vi "can decoder.vi"(10 "can cluster":T1 {"identifier" format="%03x"}, 11 "name":string="Prius") -> ()   [LabVIEW 2015]
uses:
  rio_Global.vi
panel:
  out "payload 2":u8[](array[numeric])
  out "payload":u8[](array[numeric])
  in  "sortbyID":bool
  in  "clear":bool
  out "can_log":u32[][](array[numeric]) format="%02x"
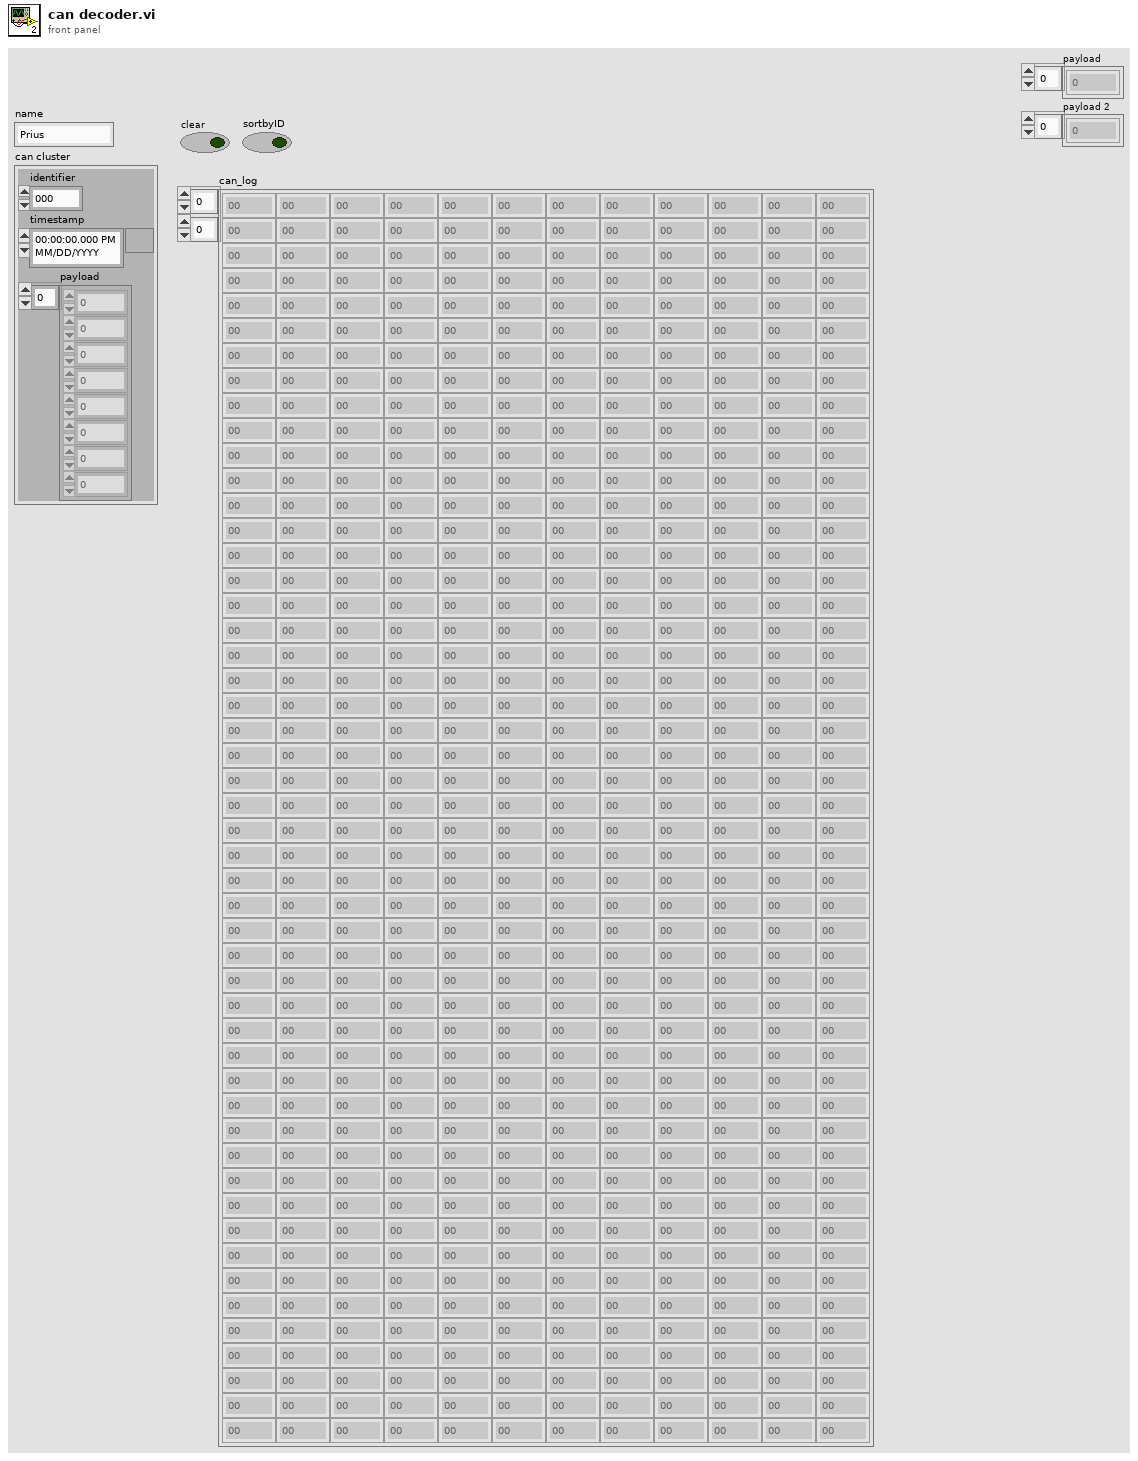
[diagram p1: front panel]
types:
  T1 = cluster{"identifier":u32, "timestamp":timestamp, "payload":u8[]}
  T2 = cluster{"identifier":u32, "identifier":u32, "identifier":u32, "identifier":u32, "identifier":u32, "identifier":u32, "identifier":u32, "identifier":u32, "identifier":u32, "identifier":u32, "identifier":u32}[]
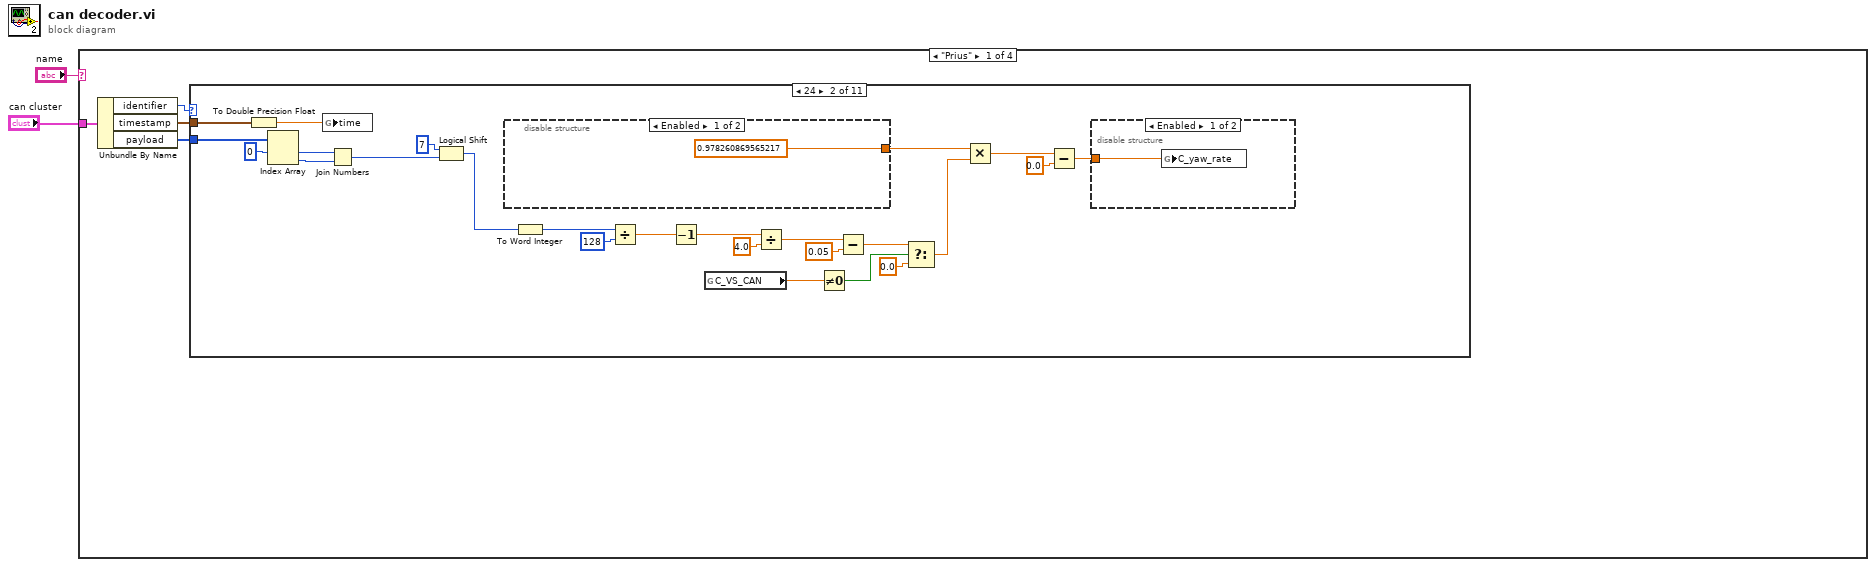
[diagram p0: block diagram]
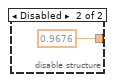
[diagram p3: hidden frame]
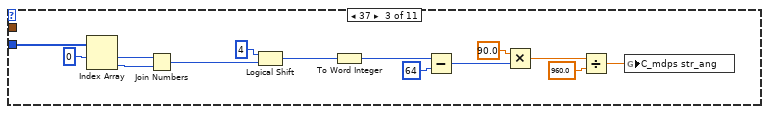
[diagram p5: hidden frame]
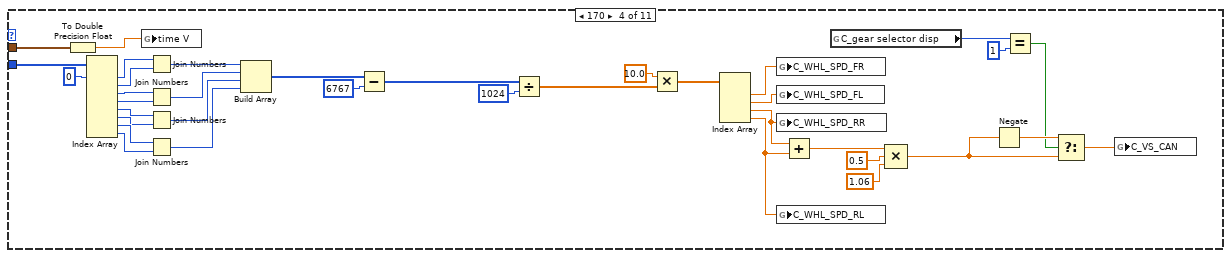
[diagram p6: hidden frame]
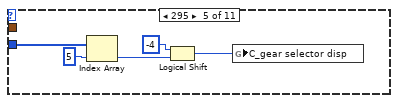
[diagram p7: hidden frame]
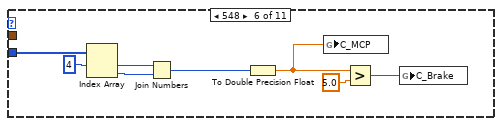
[diagram p8: hidden frame]
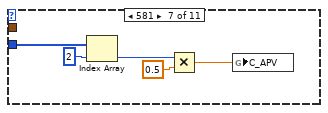
[diagram p9: hidden frame]
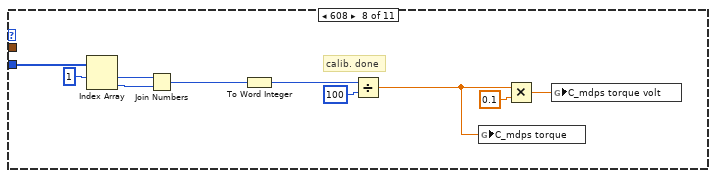
[diagram p10: hidden frame]
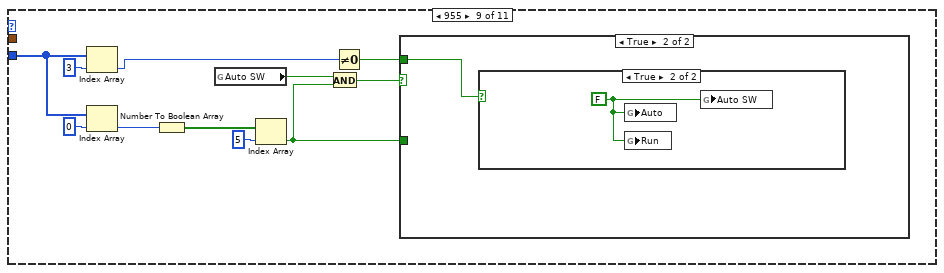
[diagram p11: hidden frame]
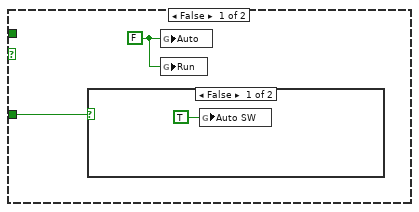
[diagram p12: hidden frame]
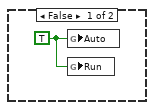
[diagram p14: hidden frame]
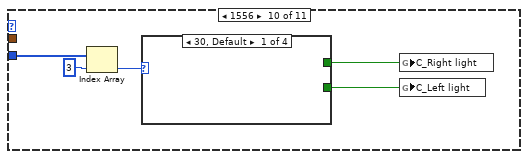
[diagram p15: hidden frame]
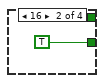
[diagram p16: hidden frame]
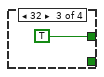
[diagram p17: hidden frame]
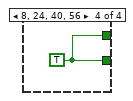
[diagram p18: hidden frame]
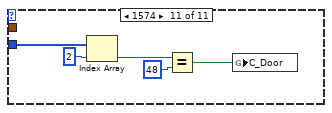
[diagram p19: hidden frame]
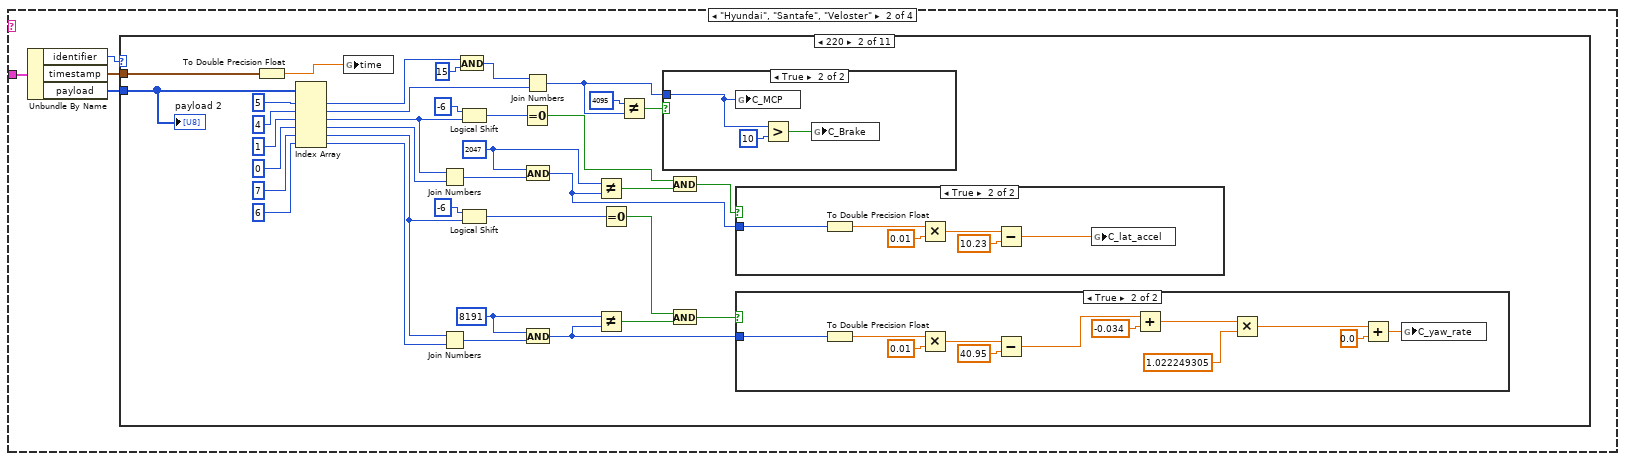
[diagram p20: hidden frame]
diagram:
  n1 = case shown="\"Prius\"" "name" {
    tunnel: "can cluster" -> [w6 w146 w412 w617]
    frame "Prius" {
      n2 = Unbundle By Name(w6) -> ("identifier"=w5:u32, "timestamp"=w4:timestamp, "payload"=w3:u8[])
      n3 = case shown="24" w5 {
        tunnel: w3 -> [_ w25 w41 w65 w89 w97 w102 w112 w115 w134 w142]
        tunnel: w4 -> [_ w22 _ w50 _ _ _ _ _ _ _]
        frame 0, Default {
        }
        frame 36 {
          n4 = To Double Precision Float(number=w22) -> (double precision float=w23:dbl)
          n5 = Index Array(array=w25, index #1=0 ("index")) -> (element #1=w27:u8, element #2=w19:u8)  [unwired: 1 in]
          n6 = global write "rio_Global.vi" "time"(w23) -> ()
          n7 = Join Numbers(hi=w27, lo=w19) -> ((hi.lo)=w18:u16)
          n8 = Logical Shift(y=i16 7, x=w18) -> (x << y=w31:u16)
          n9 = disable-structure shown="Enabled" {
            disable-tunnel: [0.978260869565217 ("x") 0.9676 ("x")] -> w8
            frame Enabled {
            }
            frame Disabled {
            }
          }
          n10 = To Word Integer(number=w31) -> (16bit integer=w30:i16)
          n11 = Divide(x=w30, y=i16 128) -> (x/y=w17:dbl)
          n12 = Decrement(x=w17) -> (x-1=w16:dbl)
          n13 = global read "rio_Global.vi" "C_VS_CAN"() -> (w13:dbl)
          n14 = Divide(x=w16, y=4.0) -> (x/y=w15:dbl)
          n15 = Not Equal To 0?(x=w13) -> (x != 0?=w12:bool)
          n16 = Subtract(x=w15, y=0.05) -> (x-y=w11:dbl)
          n17 = Select(t=w11, s=w12, f=0.0) -> (s? t:f=w9:dbl)
          n18 = Multiply(x=w8, y=w9) -> (x*y=w7:dbl)
          n19 = Subtract(x=w7, y=0.0) -> (x-y=w20:dbl)
          n20 = disable-structure shown="Enabled" {
            disable-tunnel: w20 -> [w34 _]
            frame Enabled {
              n21 = global write "rio_Global.vi" "C_yaw_rate"(w34) -> ()
            }
            frame Disabled {
            }
          }
        }
        frame 37 {
          n22 = Index Array(array=w41, index #1=0 ("index")) -> (element #1=w43:u8, element #2=w44:u8)  [unwired: 1 in]
          n23 = Join Numbers(hi=w43, lo=w44) -> ((hi.lo)=w45:u16)
          n24 = Logical Shift(y=i16 4, x=w45) -> (x << y=w47:u16)
          n25 = To Word Integer(number=w47) -> (16bit integer=w38:i16)
          n26 = Subtract(x=w38, y=i16 64) -> (x-y=w37:i16)
          n27 = Multiply(x=90.0, y=w37) -> (x*y=w39:dbl)
          n28 = Divide(x=w39, y=960.0) -> (x/y=w35:dbl)
          n29 = global write "rio_Global.vi" "C_mdps str_ang"(w35) -> ()
        }
        frame 170 {
          n30 = To Double Precision Float(number=w50) -> (double precision float=w49:dbl)
          n31 = Index Array(array=w65, index #1=0 ("index")) -> (element #1=w67:u8, element #2=w68:u8, element #3=w74:u8, element #4=w75:u8, element #5=w76:u8, element #6=w77:u8, element #7=w78:u8, element #8=w79:u8)  [unwired: 7 in]
          n32 = global write "rio_Global.vi" "time V"(w49) -> ()
          n33 = Join Numbers(hi=w67, lo=w68) -> ((hi.lo)=w80:u16)
          n34 = Join Numbers(hi=w74, lo=w75) -> ((hi.lo)=w81:u16)
          n35 = Join Numbers(hi=w76, lo=w77) -> ((hi.lo)=w82:u16)
          n36 = Join Numbers(hi=w78, lo=w79) -> ((hi.lo)=w83:u16)
          n37 = Build Array(w80, w81, w82, w83) -> (w84:u16[])
          n38 = Subtract(x=w84, y=u16 6767) -> (x-y=w70:u16[])
          n39 = Divide(x=w70, y=u16 1024) -> (x/y=w72:dbl[])
          n40 = Multiply(x=10.0, y=w72) -> (x*y=w64:dbl[])
          n41 = Index Array(array=w64) -> (element #1=w56:dbl, element #2=w57:dbl, element #3=w53:dbl, element #4=w52:dbl)  [unwired: 4 in]
          n42 = global write "rio_Global.vi" "C_WHL_SPD_FR"(w56) -> ()
          n43 = global write "rio_Global.vi" "C_WHL_SPD_FL"(w57) -> ()
          n44 = global write "rio_Global.vi" "C_WHL_SPD_RR"(w53) -> ()
          n45 = global write "rio_Global.vi" "C_WHL_SPD_RL"(w52) -> ()
          n46 = Add(x=w53, y=w52) -> (x+y=w63:dbl)
          n47 = global read "rio_Global.vi" "C_gear selector disp"() -> (w55:u8)
          n48 = Compound Arithmetic op=MULTIPLY(w63, 0.5 ("y"), 1.06 ("value")) -> (w58:dbl)
          n49 = Negate(x=w58) -> (-x=w61:dbl)
          n50 = Equal?(x=w55, y=u8 1) -> (x = y?=w60:bool)
          n51 = Select(t=w61, s=w60, f=w58) -> (s? t:f=w54:dbl)
          n52 = global write "rio_Global.vi" "C_VS_CAN"(w54) -> ()
        }
        frame 295 {
          n53 = Index Array(array=w89, index=5) -> (element=w86:u8)
          n54 = Logical Shift(y=i16 -4, x=w86) -> (x << y=w85:u8)
          n55 = global write "rio_Global.vi" "C_gear selector disp"(w85) -> ()
        }
        frame 548 {
          n56 = Index Array(array=w97, index #1=4 ("index")) -> (element #1=w95:u8, element #2=w94:u8)  [unwired: 1 in]
          n57 = Join Numbers(hi=w95, lo=w94) -> ((hi.lo)=w93:u16)
          n58 = To Double Precision Float(number=w93) -> (double precision float=w91:dbl)
          n59 = global write "rio_Global.vi" "C_MCP"(w91) -> ()
          n60 = Greater?(x=w91, y=5.0) -> (0:w90:bool)
          n61 = global write "rio_Global.vi" "C_Brake"(w90) -> ()
        }
        frame 581 {
          n62 = Index Array(array=w102, index=2) -> (element=w100:u8)
          n63 = Multiply(x=w100, y=0.5) -> (x*y=w98:dbl)
          n64 = global write "rio_Global.vi" "C_APV"(w98) -> ()
        }
        frame 608 {
          # "calib. done"
          n65 = Index Array(array=w112, index #1=1 ("index")) -> (element #1=w110:u8, element #2=w109:u8)  [unwired: 1 in]
          n66 = Join Numbers(hi=w110, lo=w109) -> ((hi.lo)=w108:u16)
          n67 = To Word Integer(number=w108) -> (16bit integer=w106:i16)
          n68 = Divide(x=w106, y=i16 100) -> (x/y=w104:dbl)
          n69 = global write "rio_Global.vi" "C_mdps torque"(w104) -> ()
          n70 = Multiply(x=w104, y=0.1) -> (x*y=w103:dbl)
          n71 = global write "rio_Global.vi" "C_mdps torque volt"(w103) -> ()
        }
        frame 955 {
          n72 = Index Array(array=w115, index=3) -> (element=w113:u8)
          n73 = Index Array(array=w115, index=0) -> (element=w122:u8)
          n74 = Number To Boolean Array(number=w122) -> (Boolean array=w121:bool[])
          n75 = global read "rio_Global.vi" "Auto SW"() -> (w119:bool)
          n76 = Index Array(array=w121, index=5) -> (element=w117:bool)
          n77 = And(x=w119, y=w117) -> (x .and. y?=w118:bool)
          n78 = Not Equal To 0?(x=w113) -> (x != 0?=w116:bool)
          n79 = case shown="True" w118 {
            tunnel: w116 -> [_ w127]
            tunnel: w117 -> [w125 _]
            frame False {
              w124 = FALSE ("Auto SW")
              n80 = case shown="False" w125 {
                frame False {
                  n81 = global write "rio_Global.vi" "Auto SW"(TRUE ("Auto SW")) -> ()
                }
                frame True {
                }
              }
              n82 = global write "rio_Global.vi" "Auto"(w124) -> ()
              n83 = global write "rio_Global.vi" "Run"(w124) -> ()
            }
            frame True {
              n84 = case shown="True" w127 {
                frame False {
                  w128 = TRUE ("Auto")
                  n85 = global write "rio_Global.vi" "Auto"(w128) -> ()
                  n86 = global write "rio_Global.vi" "Run"(w128) -> ()
                }
                frame True {
                  w129 = FALSE ("Auto SW")
                  n87 = global write "rio_Global.vi" "Auto"(w129) -> ()
                  n88 = global write "rio_Global.vi" "Run"(w129) -> ()
                  n89 = global write "rio_Global.vi" "Auto SW"(w129) -> ()
                }
              }
            }
          }
        }
        frame 1556 {
          n90 = Index Array(array=w134, index=3) -> (element=w132:u8)
          n91 = case shown="30, Default" w132 {
            tunnel: [_ TRUE _ w137] -> w131
            tunnel: [_ _ TRUE w137] -> w130
            frame 48, Default {
            }
            frame 16 {
            }
            frame 32 {
            }
            frame 8, 24, 40, 56 {
              w137 = TRUE
            }
          }
          n92 = global write "rio_Global.vi" "C_Right light"(w130) -> ()
          n93 = global write "rio_Global.vi" "C_Left light"(w131) -> ()
        }
        frame 1574 {
          n94 = Index Array(array=w142, index=2) -> (element=w140:u8)
          n95 = Equal?(x=w140, y=u8 48) -> (x = y?=w138:bool)
          n96 = global write "rio_Global.vi" "C_Door"(w138) -> ()
        }
      }
    }
    frame "Hyundai", "Santafe", "Veloster" {
      n97 = Unbundle By Name(w146) -> ("identifier"=w145:u32, "timestamp"=w144:timestamp, "payload"=w143:u8[])
      n98 = case shown="220" w145 {
        tunnel: w143 -> [_ w147 w205 w223 w244 w299 w303 w305 w314 w368 w392]
        tunnel: w144 -> [_ w182 _ _ _ _ _ _ w312 _ _]
        frame 0, Default {
        }
        frame 544 {
          w151 = u16 8191
          w158 = u16 2047
          n99 = To Double Precision Float(number=w182) -> (double precision float=w181:dbl)
          n100 = Index Array(array=w147, index #1=5 ("index"), index #2=4 ("index"), index #3=1 ("index"), index #4=0 ("index"), index #5=7 ("index"), index #6=6 ("index")) -> (element #1=w174:u8, element #2=w173:u8, element #3=w172:u8, element #4=w171:u8, element #5=w170:u8, element #6=w169:u8)
          n101 = global write "rio_Global.vi" "time"(w181) -> ()
          n102 = Join Numbers(hi=w172, lo=w171) -> ((hi.lo)=w159:u16)
          n103 = Join Numbers(hi=w170, lo=w169) -> ((hi.lo)=w150:u16)
          n104 = And(x=w174, y=u8 15) -> (x .and. y?=w167:u8)
          n105 = Logical Shift(y=i16 -6, x=w172) -> (x << y=w161:u8)
          n106 = Logical Shift(y=i16 -6, x=w170) -> (x << y=w154:u8)
          n107 = Equal To 0?(x=w161) -> (x = 0?=w162:bool)
          n108 = Join Numbers(hi=w167, lo=w173) -> ((hi.lo)=w164:u16)
          n109 = And(x=w158, y=w159) -> (x .and. y?=w157:u16)
          n110 = And(x=w151, y=w150) -> (x .and. y?=w149:u16)
          n111 = Not Equal?(x=w158, y=w157) -> (x != y?=w163:bool)
          n112 = Not Equal?(x=w151, y=w149) -> (x != y?=w152:bool)
          n113 = Equal To 0?(x=w154) -> (x = 0?=w153:bool)
          n114 = Not Equal?(x=u16 4095, y=w164) -> (x != y?=w165:bool)
          n115 = case shown="True" w165 {
            tunnel: w164 -> [_ w201]
            frame False {
            }
            frame True {
              n116 = global write "rio_Global.vi" "C_MCP"(w201) -> ()
              n117 = Greater?(x=w201, y=u16 10) -> (0:w203:bool)
              n118 = global write "rio_Global.vi" "C_Brake"(w203) -> ()
            }
          }
          n119 = And(x=w162, y=w163) -> (x .and. y?=w156:bool)
          n120 = And(x=w153, y=w152) -> (x .and. y?=w148:bool)
          n121 = case shown="True" w156 {
            tunnel: w157 -> [_ w200]
            frame False {
            }
            frame True {
              n122 = To Double Precision Float(number=w200) -> (double precision float=w199:dbl)
              n123 = Multiply(x=w199, y=0.01) -> (x*y=w197:dbl)
              n124 = Subtract(x=w197, y=10.23) -> (x-y=w195:dbl)
              n125 = global write "rio_Global.vi" "C_lat_accel"(w195) -> ()
            }
          }
          n126 = case shown="True" w148 {
            tunnel: w149 -> [_ w194]
            frame False {
            }
            frame True {
              n127 = To Double Precision Float(number=w194) -> (double precision float=w193:dbl)
              n128 = Multiply(x=w193, y=0.01) -> (x*y=w191:dbl)
              n129 = Subtract(x=w191, y=40.95) -> (x-y=w184:dbl)
              n130 = Add(x=w184, y=-0.034) -> (x+y=w183:dbl)
              n131 = Multiply(x=w183, y=1.022249305) -> (x*y=w187:dbl)
              n132 = Add(x=w187, y=0.0) -> (x+y=w186:dbl)
              n133 = global write "rio_Global.vi" "C_yaw_rate"(w186) -> ()
            }
          }
          "payload 2" <- w147
        }
        frame 608 {
          n134 = global read "rio_Global.vi" "Car_name"() -> (w204:string)
          n135 = Equal?(x=w204, y="Santafe") -> (x = y?=w206:bool)
          n136 = case shown="True" w206 {
            tunnel: w205 -> [_ w216]
            frame False {
            }
            frame True {
              n137 = Index Array(array=w216, index=3) -> (element=w214:u8)
              n138 = Number To Boolean Array(number=w214) -> (Boolean array=w213:bool[])
              n139 = global read "rio_Global.vi" "Auto SW"() -> (w210:bool)
              n140 = Index Array(array=w213, index #1=1 ("index")) -> (element #1=w208:bool, element #2=w211:bool)  [unwired: 1 in]
              n141 = And(x=w210, y=w208) -> (x .and. y?=w209:bool)
              n142 = case shown="False" w209 {
                tunnel: w211 -> [_ w220]
                tunnel: w208 -> [w218 _]
                frame False {
                  w217 = FALSE ("Auto SW")
                  n143 = case shown="False" w218 {
                    frame False {
                      n144 = global write "rio_Global.vi" "Auto SW"(TRUE ("Auto SW")) -> ()
                    }
                    frame True {
                    }
                  }
                  n145 = global write "rio_Global.vi" "Auto"(w217) -> ()
                  n146 = global write "rio_Global.vi" "Run"(w217) -> ()
                }
                frame True {
                  n147 = case shown="True" w220 {
                    frame False {
                      w221 = TRUE ("Auto")
                      n148 = global write "rio_Global.vi" "Auto"(w221) -> ()
                      n149 = global write "rio_Global.vi" "Run"(w221) -> ()
                    }
                    frame True {
                      w222 = FALSE ("Auto SW")
                      n150 = global write "rio_Global.vi" "Auto"(w222) -> ()
                      n151 = global write "rio_Global.vi" "Run"(w222) -> ()
                      n152 = global write "rio_Global.vi" "Auto SW"(w222) -> ()
                    }
                  }
                }
              }
            }
          }
        }
        frame 809 {
          n153 = Index Array(array=w223, index #1=5 ("index"), index #2=6 ("index")) -> (element #1=w226:u8, element #2=w229:u8)
          n154 = Not Equal?(x=w226, y=u8 255 ("x")) -> (x != y?=w230:bool)
          n155 = Not Equal?(x=w229, y=u8 255 ("x")) -> (x != y?=w231:bool)
          n156 = case shown="True" w230 {
            tunnel: w226 -> [_ w243]
            frame False {
            }
            frame True {
              n157 = Subtract(x=w243, y=u8 32) -> (x-y=w241:u8)
              n158 = To Double Precision Float(number=w241) -> (double precision float=w240:dbl)
              n159 = Multiply(x=w240, y=100.0) -> (x*y=w238:dbl)
              n160 = Divide(x=w238, y=213.0) -> (x/y=w236:dbl)
              n161 = global write "rio_Global.vi" "C_tps"(w236) -> ()
            }
          }
          n162 = case shown="True" w231 {
            tunnel: w229 -> [_ w235]
            frame False {
            }
            frame True {
              n163 = To Double Precision Float(number=w235) -> (double precision float=w234:dbl)
              n164 = Multiply(x=w234, y=0.3906) -> (x*y=w233:dbl)
              n165 = global write "rio_Global.vi" "C_APV"(w233) -> ()
            }
          }
        }
        frame 914 {
          n166 = Array Subset(array=w244, index=0, length=7) -> (w248:u8[])
          n167 = Index Array(array=w244, index #1=7 ("index"), index #2=2 ("index"), index #3=1 ("index"), index #4=4 ("index"), index #5=3 ("index")) -> (element #1=w245:u8, element #2=w256:u8, element #3=w255:u8, element #4=w252:u8, element #5=w251:u8)
          n168 = Add Array Elements(numeric array=w248) -> (sum=w246:u8)
          n169 = Equal?(x=w246, y=w245) -> (x = y?=w247:bool)
          n170 = case shown="True" w247 {
            tunnel: w256 -> [_ w270]
            tunnel: w255 -> [_ w269]
            tunnel: w252 -> [_ w266]
            tunnel: w251 -> [_ w265]
            frame False {
            }
            frame True {
              w261 = u16 4095 ("y")
              n171 = Join Numbers(hi=w270, lo=w269) -> ((hi.lo)=w262:u16)
              n172 = Join Numbers(hi=w266, lo=w265) -> ((hi.lo)=w267:u16)
              n173 = And(x=w261, y=w262) -> (x .and. y?=w260:u16)
              n174 = Not Equal?(x=w267, y=u16 32767 ("x")) -> (x != y?=w263:bool)
              n175 = Not Equal?(x=w261, y=w260) -> (x != y?=w264:bool)
              n176 = case shown="True" w264 {
                tunnel: w260 -> [_ w283]
                frame False {
                }
                frame True {
                  n177 = To Double Precision Float(number=w283) -> (double precision float=w282:dbl)
                  n178 = Subtract(x=w282, y=2048.0) -> (x-y=w281:dbl)
                  n179 = Multiply(x=w281, y=0.01) -> (x*y=w280:dbl)
                  n180 = global write "rio_Global.vi" "C_mdps torque"(w280) -> ()
                }
              }
              n181 = case shown="True" w263 {
                tunnel: w267 -> [_ w277]
                frame False {
                }
                frame True {
                  n182 = To Double Precision Float(number=w277) -> (double precision float=w274:dbl)
                  n183 = Subtract(x=w274, y=65536.0) -> (x-y=w275:dbl)
                  n184 = Greater?(x=w274, y=32767.0 ("x")) -> (0:w278:bool)
                  n185 = Select(t=w275, s=w278, f=w274) -> (s? t:f=w273:dbl)
                  n186 = Multiply(x=w273, y=0.1) -> (x*y=w271:dbl)
                  n187 = global write "rio_Global.vi" "C_mdps str_ang"(w271) -> ()
                }
              }
            }
          }
        }
        frame 688 {
          n188 = Index Array(array=w299, index #1=1 ("index"), index #2=0 ("index")) -> (element #1=w296:u8, element #2=w295:u8)
          n189 = Join Numbers(hi=w296, lo=w295) -> ((hi.lo)=w287:u16)
          n190 = To Long Integer(number=w287) -> (32bit integer=w286:i32)
          n191 = Greater?(x=w286, y=32767) -> (0:w293:bool)
          n192 = Subtract(x=w286, y=65535) -> (x-y=w291:i32)
          n193 = Select(t=w291, s=w293, f=w286) -> (s? t:f=w290:i32)
          n194 = Multiply(x=w290, y=0.1) -> (x*y=w288:dbl)
          n195 = disable-structure shown="Disabled" {
            disable-tunnel: w288 -> [w300 _]
            frame Disabled {
              n196 = global write "rio_Global.vi" "C_mdps str_ang"(w300) -> ()
            }
            frame Enabled {
            }
          }
        }
        frame 790 {
          n197 = Index Array(array=w303, index=6) -> (element=w301:u8)
          n198 = disable-structure shown="Disabled" {
            disable-tunnel: w301 -> [w304 _]
            frame Disabled {
              n199 = global write "rio_Global.vi" "C_VS_CAN"(w304) -> ()
            }
            frame Enabled {
            }
          }
        }
        frame 1087 {
          w308 = u8 15 ("y")
          n200 = Index Array(array=w305, index=1) -> (element=w307:u8)
          n201 = And(x=w307, y=w308) -> (x .and. y?=w309:u8)
          n202 = Not Equal?(x=w309, y=w308) -> (x != y?=w310:bool)
          n203 = case shown="True" w310 {
            tunnel: w309 -> [_ w311]
            frame False {
            }
            frame True {
              n204 = global write "rio_Global.vi" "C_gear selector disp"(w311) -> ()
            }
          }
        }
        frame 1200 {
          w318 = u16 16383 ("x")
          w331 = u16 16383 ("x")
          n205 = To Double Precision Float(number=w312) -> (double precision float=w313:dbl)
          n206 = Index Array(array=w314, index #1=1 ("index"), index #2=0 ("index"), index #3=3 ("index"), index #4=2 ("index"), index #5=5 ("index"), index #6=4 ("index"), index #7=7 ("index"), index #8=6 ("index")) -> (element #1=w323:u8, element #2=w322:u8, element #3=w321:u8, element #4=w320:u8, element #5=w341:u8, element #6=w340:u8, element #7=w336:u8, element #8=w335:u8)
          n207 = global write "rio_Global.vi" "time V"(w313) -> ()
          n208 = Join Numbers(hi=w323, lo=w322) -> ((hi.lo)=w319:u16)
          n209 = Join Numbers(hi=w321, lo=w320) -> ((hi.lo)=w317:u16)
          n210 = Join Numbers(hi=w341, lo=w340) -> ((hi.lo)=w339:u16)
          n211 = Join Numbers(hi=w336, lo=w335) -> ((hi.lo)=w332:u16)
          n212 = And(x=w319, y=w318) -> (x .and. y?=w316:u16)
          n213 = And(x=w318, y=w317) -> (x .and. y?=w315:u16)
          n214 = And(x=w339, y=w331) -> (x .and. y?=w330:u16)
          n215 = And(x=w331, y=w332) -> (x .and. y?=w329:u16)
          n216 = Not Equal?(x=w330, y=w331) -> (x != y?=w334:bool)
          n217 = Not Equal?(x=w331, y=w329) -> (x != y?=w333:bool)
          n218 = And(x=w334, y=w333) -> (x .and. y?=w328:bool)
          n219 = case shown="True" w328 {
            tunnel: w330 -> [_ w367]
            tunnel: w329 -> [_ w366]
            tunnel: w316 -> [_ w360]
            tunnel: w315 -> [_ w359]
            frame False {
            }
            frame True {
              w355 = 0.03125 ("y")
              w365 = 0.03125 ("y")
              n220 = To Double Precision Float(number=w360) -> (double precision float=w357:dbl)
              n221 = To Double Precision Float(number=w359) -> (double precision float=w354:dbl)
              n222 = To Double Precision Float(number=w367) -> (double precision float=w358:dbl)
              n223 = To Double Precision Float(number=w366) -> (double precision float=w351:dbl)
              n224 = Multiply(x=w357, y=w355) -> (x*y=w356:dbl)
              n225 = Multiply(x=w355, y=w354) -> (x*y=w353:dbl)
              n226 = Multiply(x=w358, y=w365) -> (x*y=w352:dbl)
              n227 = Multiply(x=w365, y=w351) -> (x*y=w350:dbl)
              n228 = global write "rio_Global.vi" "C_WHL_SPD_FL"(w356) -> ()
              n229 = global write "rio_Global.vi" "C_WHL_SPD_FR"(w353) -> ()
              n230 = global write "rio_Global.vi" "C_WHL_SPD_RL"(w352) -> ()
              n231 = global write "rio_Global.vi" "C_WHL_SPD_RR"(w350) -> ()
              n232 = Add(x=w352, y=w350) -> (x+y=w364:dbl)
              n233 = global read "rio_Global.vi" "C_gear selector disp"() -> (w347:u8)
              n234 = Multiply(x=w364, y=0.5) -> (x*y=w361:dbl)
              n235 = Multiply(x=w361, y=1.0) -> (x*y=w345:dbl)
              n236 = Negate(x=w345) -> (-x=w349:dbl)
              n237 = Equal?(x=w347, y=u8 7) -> (x = y?=w348:bool)
              n238 = Select(t=w349, s=w348, f=w345) -> (s? t:f=w344:dbl)
              n239 = global write "rio_Global.vi" "C_VS_CAN"(w344) -> ()
            }
          }
          "payload" <- w314
        }
        frame 1264 {
          n240 = disable-structure shown="Enabled" {
            disable-tunnel: w368 -> [w373 w377]
            frame Disabled {
              n241 = Index Array(array=w373, index=3) -> (element=w371:u8)
              n242 = case shown="8, 18, 28, 38" w371 {
                tunnel: [_ TRUE _ w376] -> w370
                tunnel: [_ _ TRUE w376] -> w369
                frame 48, Default {
                }
                frame 16 {
                }
                frame 32 {
                }
                frame 8, 24, 40, 56 {
                  w376 = TRUE
                }
              }
              n243 = global write "rio_Global.vi" "C_Right light"(w369) -> ()
              n244 = global write "rio_Global.vi" "C_Left light"(w370) -> ()
            }
            frame Enabled {
              n245 = Index Array(array=w377, index #1=7 ("index"), index #2=6 ("index"), index #3=5 ("index")) -> (element #1=w383:u8, element #2=w381:u8, element #3=w382:u8)
              n246 = Join Numbers(hi=w381, lo=w382) -> ((hi.lo)=w386:u16)
              n247 = Join Numbers(hi=u8 0, lo=w383) -> ((hi.lo)=w385:u16)
              n248 = Join Numbers(hi=w385, lo=w386) -> ((hi.lo)=w388:u32)
              n249 = Not Equal?(x=u32 16777215, y=w388) -> (x != y?=w389:bool)
              n250 = case shown="True" w389 {
                tunnel: w388 -> [_ w391]
                frame False {
                }
                frame True {
                  n251 = To Double Precision Float(number=w391) -> (double precision float=w390:dbl)
                  n252 = global write "rio_Global.vi" "C_odometer"(w390) -> ()
                }
              }
            }
          }
        }
        frame 1349 {
          n253 = disable-structure shown="Enabled" {
            disable-tunnel: w392 -> [w397 w398]
            frame Disabled {
              n254 = Index Array(array=w397, index=2) -> (element=w395:u8)
              n255 = Equal?(x=w395, y=u8 48) -> (x = y?=w393:bool)
              n256 = global write "rio_Global.vi" "C_Door"(w393) -> ()
            }
            frame Enabled {
              n257 = Index Array(array=w398, index=3) -> (element=w401:u8)
              n258 = Not Equal?(x=w401, y=u8 255 ("x")) -> (x != y?=w399:bool)
              n259 = case shown="True" w399 {
                tunnel: w401 -> [_ w408]
                frame False {
                }
                frame True {
                  n260 = To Double Precision Float(number=w408) -> (double precision float=w407:dbl)
                  n261 = Multiply(x=26.0, y=w407) -> (x*y=w405:dbl)
                  n262 = Divide(x=w405, y=256.0) -> (x/y=w403:dbl)
                  n263 = global write "rio_Global.vi" "C_battery voltage"(w403) -> ()
                }
              }
            }
          }
        }
      }
    }
    frame "Avante" {
      n264 = Unbundle By Name(w412) -> ("identifier"=w411:u32, "timestamp"=w410:timestamp, "payload"=w409:u8[])
      n265 = case shown="220" w411 {
        tunnel: w409 -> [_ w414 w477 w513 w514 w523 w577 w604]
        tunnel: w410 -> [_ w446 _ _ _ w521 _ _]
        frame 0, Default {
        }
        frame 544 {
          w417 = u16 8191
          w422 = u16 2047
          n266 = To Double Precision Float(number=w446) -> (double precision float=w445:dbl)
          n267 = Index Array(array=w414, index #1=4 ("index"), index #2=3 ("index"), index #3=1 ("index"), index #4=0 ("index"), index #5=6 ("index"), index #6=5 ("index")) -> (element #1=w438:u8, element #2=w437:u8, element #3=w436:u8, element #4=w435:u8, element #5=w434:u8, element #6=w433:u8)
          n268 = global write "rio_Global.vi" "time"(w445) -> ()
          n269 = Join Numbers(hi=w436, lo=w435) -> ((hi.lo)=w423:u16)
          n270 = Join Numbers(hi=w434, lo=w433) -> ((hi.lo)=w416:u16)
          n271 = And(x=w438, y=u8 15) -> (x .and. y?=w431:u8)
          n272 = Logical Shift(y=i16 -6, x=w436) -> (x << y=w425:u8)
          n273 = Logical Shift(y=i16 -6, x=w434) -> (x << y=w418:u8)
          n274 = Equal To 0?(x=w418) -> ()  [unwired: 1 out]
          n275 = Join Numbers(hi=w431, lo=w437) -> ((hi.lo)=w428:u16)
          n276 = Equal To 0?(x=w425) -> (x = 0?=w426:bool)
          n277 = And(x=w422, y=w423) -> (x .and. y?=w421:u16)
          n278 = And(x=w417, y=w416) -> (x .and. y?=w415:u16)
          n279 = Not Equal?(x=w417, y=w415) -> ()  [unwired: 1 out]
          n280 = Not Equal?(x=w422, y=w421) -> (x != y?=w427:bool)
          n281 = Not Equal?(x=u16 4095, y=w428) -> (x != y?=w429:bool)
          n282 = case shown="True" w429 {
            tunnel: w428 -> [_ w470]
            frame False {
            }
            frame True {
              n283 = Multiply(x=w470, y=0.1) -> (x*y=w469:dbl)
              n284 = global write "rio_Global.vi" "C_MCP"(w469) -> ()
            }
          }
          n285 = case shown="True" TRUE {
            tunnel: w415 -> [_ w453]
            frame False {
            }
            frame True {
              n286 = To Double Precision Float(number=w453) -> (double precision float=w452:dbl)
              n287 = Multiply(x=w452, y=0.01) -> (x*y=w450:dbl)
              n288 = Subtract(x=w450, y=40.95) -> (x-y=w447:dbl)
              n289 = disable-structure shown="Enabled" {
                disable-tunnel: [w457 w461] -> w448
                disable-tunnel: w447 -> [w455 w461]
                frame Disabled {
                  n290 = Add(x=w455, y=-0.034) -> (x+y=w454:dbl)
                  n291 = Multiply(x=w454, y=1.045) -> (x*y=w458:dbl)
                  n292 = Add(x=w458, y=0.0) -> (x+y=w457:dbl)
                }
                frame Enabled {
                }
              }
              n293 = global write "rio_Global.vi" "C_yaw_rate"(w448) -> ()
            }
          }
          n294 = And(x=w426, y=w427) -> (x .and. y?=w420:bool)
          n295 = case shown="True" w420 {
            tunnel: w421 -> [_ w467]
            frame False {
            }
            frame True {
              n296 = To Double Precision Float(number=w467) -> (double precision float=w466:dbl)
              n297 = Multiply(x=w466, y=0.01) -> (x*y=w464:dbl)
              n298 = Subtract(x=w464, y=10.23) -> (x-y=w462:dbl)
              n299 = global write "rio_Global.vi" "C_lat_accel"(w462) -> ()
            }
          }
        }
        frame 809 {
          n300 = Index Array(array=w477, index #1=4 ("index"), index #2=5 ("index"), index #3=6 ("index")) -> (element #1=w475:u8, element #2=w480:u8, element #3=w483:u8)
          n301 = And(x=u8 3, y=w475) -> (x .and. y?=w473:u8)
          n302 = Not Equal?(x=w480, y=u8 255 ("x")) -> (x != y?=w484:bool)
          n303 = Not Equal?(x=w483, y=u8 255 ("x")) -> (x != y?=w485:bool)
          n304 = case shown="True" w484 {
            tunnel: w480 -> [_ w497]
            frame False {
            }
            frame True {
              n305 = Subtract(x=w497, y=u8 32) -> (x-y=w495:u8)
              n306 = To Double Precision Float(number=w495) -> (double precision float=w494:dbl)
              n307 = Multiply(x=w494, y=100.0) -> (x*y=w492:dbl)
              n308 = Divide(x=w492, y=213.0) -> (x/y=w490:dbl)
              n309 = global write "rio_Global.vi" "C_tps"(w490) -> ()
            }
          }
          n310 = case shown="True" w485 {
            tunnel: w483 -> [_ w489]
            frame False {
            }
            frame True {
              n311 = To Double Precision Float(number=w489) -> (double precision float=w488:dbl)
              n312 = Multiply(x=w488, y=0.3906) -> (x*y=w487:dbl)
              n313 = global write "rio_Global.vi" "C_APV"(w487) -> ()
            }
          }
          n314 = Equal?(x=u8 2, y=w473) -> (x = y?=w471:bool)
          n315 = global write "rio_Global.vi" "C_Brake"(w471) -> ()
        }
        frame 688 {
          n316 = Index Array(array=w513, index #1=1 ("index"), index #2=0 ("index"), index #3=2 ("index"), index #4=4 ("index")) -> (element #1=w510:u8, element #2=w509:u8)  [unwired: 2 in, 4 out]
          n317 = Join Numbers(hi=w510, lo=w509) -> ((hi.lo)=w501:u16)
          n318 = To Long Integer(number=w501) -> (32bit integer=w500:i32)
          n319 = Greater?(x=w500, y=32767) -> (0:w507:bool)
          n320 = Subtract(x=w500, y=65535) -> (x-y=w505:i32)
          n321 = Select(t=w505, s=w507, f=w500) -> (s? t:f=w504:i32)
          n322 = Multiply(x=w504, y=0.1) -> (x*y=w502:dbl)
          n323 = global write "rio_Global.vi" "C_mdps str_ang"(w502) -> ()
        }
        frame 273 {
          w517 = u8 15 ("y")
          n324 = Index Array(array=w514, index=1) -> (element=w516:u8)
          n325 = And(x=w516, y=w517) -> (x .and. y?=w518:u8)
          n326 = Not Equal?(x=w518, y=w517) -> (x != y?=w519:bool)
          n327 = case shown="True" w519 {
            tunnel: w518 -> [_ w520]
            frame False {
            }
            frame True {
              n328 = global write "rio_Global.vi" "C_gear selector disp"(w520) -> ()
            }
          }
        }
        frame 902 {
          w527 = u16 16383 ("x")
          w540 = u16 16383 ("x")
          n329 = To Double Precision Float(number=w521) -> (double precision float=w522:dbl)
          n330 = Index Array(array=w523, index #1=1 ("index"), index #2=0 ("index"), index #3=3 ("index"), index #4=2 ("index"), index #5=5 ("index"), index #6=4 ("index"), index #7=7 ("index"), index #8=6 ("index")) -> (element #1=w532:u8, element #2=w531:u8, element #3=w530:u8, element #4=w529:u8, element #5=w550:u8, element #6=w549:u8, element #7=w545:u8, element #8=w544:u8)
          n331 = global write "rio_Global.vi" "time V"(w522) -> ()
          n332 = Join Numbers(hi=w532, lo=w531) -> ((hi.lo)=w528:u16)
          n333 = Join Numbers(hi=w530, lo=w529) -> ((hi.lo)=w526:u16)
          n334 = Join Numbers(hi=w550, lo=w549) -> ((hi.lo)=w548:u16)
          n335 = Join Numbers(hi=w545, lo=w544) -> ((hi.lo)=w541:u16)
          n336 = And(x=w528, y=w527) -> (x .and. y?=w525:u16)
          n337 = And(x=w527, y=w526) -> (x .and. y?=w524:u16)
          n338 = And(x=w548, y=w540) -> (x .and. y?=w539:u16)
          n339 = And(x=w540, y=w541) -> (x .and. y?=w538:u16)
          n340 = Not Equal?(x=w539, y=w540) -> (x != y?=w543:bool)
          n341 = Not Equal?(x=w540, y=w538) -> (x != y?=w542:bool)
          n342 = And(x=w543, y=w542) -> (x .and. y?=w537:bool)
          n343 = case shown="True" w537 {
            tunnel: w539 -> [_ w576]
            tunnel: w538 -> [_ w575]
            tunnel: w525 -> [_ w569]
            tunnel: w524 -> [_ w568]
            frame False {
            }
            frame True {
              w564 = 0.03125 ("y")
              w574 = 0.03125 ("y")
              n344 = To Double Precision Float(number=w569) -> (double precision float=w566:dbl)
              n345 = To Double Precision Float(number=w568) -> (double precision float=w563:dbl)
              n346 = To Double Precision Float(number=w576) -> (double precision float=w567:dbl)
              n347 = To Double Precision Float(number=w575) -> (double precision float=w560:dbl)
              n348 = Multiply(x=w566, y=w564) -> (x*y=w565:dbl)
              n349 = Multiply(x=w564, y=w563) -> (x*y=w562:dbl)
              n350 = Multiply(x=w567, y=w574) -> (x*y=w561:dbl)
              n351 = Multiply(x=w574, y=w560) -> (x*y=w559:dbl)
              n352 = global write "rio_Global.vi" "C_WHL_SPD_FL"(w565) -> ()
              n353 = global write "rio_Global.vi" "C_WHL_SPD_FR"(w562) -> ()
              n354 = global write "rio_Global.vi" "C_WHL_SPD_RL"(w561) -> ()
              n355 = global write "rio_Global.vi" "C_WHL_SPD_RR"(w559) -> ()
              n356 = Add(x=w561, y=w559) -> (x+y=w573:dbl)
              n357 = global read "rio_Global.vi" "C_gear selector disp"() -> (w556:u8)
              n358 = Multiply(x=w573, y=0.5) -> (x*y=w570:dbl)
              n359 = Multiply(x=w570, y=1.0) -> (x*y=w554:dbl)
              n360 = Negate(x=w554) -> (-x=w558:dbl)
              n361 = Equal?(x=w556, y=u8 7) -> (x = y?=w557:bool)
              n362 = Select(t=w558, s=w557, f=w554) -> (s? t:f=w553:dbl)
              n363 = global write "rio_Global.vi" "C_VS_CAN"(w553) -> ()
            }
          }
        }
        frame 1349 {
          n364 = disable-structure shown="Enabled" {
            disable-tunnel: w577 -> [w582 w583]
            frame Disabled {
              n365 = Index Array(array=w582, index=2) -> (element=w580:u8)
              n366 = Equal?(x=w580, y=u8 48) -> (x = y?=w578:bool)
              n367 = global write "rio_Global.vi" "C_Door"(w578) -> ()
            }
            frame Enabled {
              n368 = Index Array(array=w583, index=3) -> (element=w586:u8)
              n369 = Not Equal?(x=w586, y=u8 255 ("x")) -> (x != y?=w584:bool)
              n370 = case shown="True" w584 {
                tunnel: w586 -> [_ w593]
                frame False {
                }
                frame True {
                  n371 = To Double Precision Float(number=w593) -> (double precision float=w592:dbl)
                  n372 = Multiply(x=26.0, y=w592) -> (x*y=w590:dbl)
                  n373 = Divide(x=w590, y=256.0) -> (x/y=w588:dbl)
                  n374 = global write "rio_Global.vi" "C_battery voltage"(w588) -> ()
                }
              }
            }
          }
        }
        frame 1345 {
          w595 = u8 64 ("y")
          w599 = u8 8 ("y")
          n375 = Index Array(array=w604, index #1=2 ("index"), index #2=7 ("index")) -> (element #1=w601:u8, element #2=w596:u8)
          n376 = And(x=w601, y=w599) -> (x .and. y?=w600:u8)
          n377 = And(x=w596, y=w595) -> (x .and. y?=w597:u8)
          n378 = Equal?(x=w600, y=w599) -> (x = y?=w598:bool)
          n379 = Equal?(x=w597, y=w595) -> (x = y?=w594:bool)
          n380 = global write "rio_Global.vi" "C_Left light"(w598) -> ()
          n381 = global write "rio_Global.vi" "C_Right light"(w594) -> ()
        }
      }
    }
    frame "unknown", Default {
      n382 = Unbundle By Name(w617) -> ("identifier"=w607:u32, "timestamp"=w605:timestamp, "payload"=w606:u8[])
      n383 = To Unsigned Long Integer(number=w605) -> (unsigned 32bit integer=w615:u32)
      n384 = To Unsigned Long Integer(number=w606) -> (unsigned 32bit integer=w616:u32[])
      n385 = First Call?() -> (First Call?: T/F=w613:bool)
      n386 = Build Array (concatenate)(w607, w615, w616) -> (w614:u32[])
      n387 = Or(x="clear", y=w613) -> (x .or. y?=w612:bool)
      n388 = case shown="False" w612 {
        tunnel: w614 -> [w660 w678]
        tunnel: [w659 w677] -> w609
        tunnel: w607 -> [w666 _]
        frame False {
          n389 = local read "can_log"() -> (w662:u32[][])
          n390 = Index Array(array=w662, index (col)=0 ("disabled index (col)")) -> (element=w667:u32[])  [unwired: 1 in]
          n391 = Equal?(x=w666, y=w667) -> (x = y?=w663:bool[])
          n392 = Or Array Elements(Boolean array=w663) -> (logical OR=w665:bool)
          n393 = Boolean To (0,1)(Boolean=w663) -> (0, 1=w664:i16[])
          n394 = Array Max & Min(array=w664) -> (max index (indices)=w661:i32)  [unwired: 3 out]
          n395 = case shown="False" w665 {
            tunnel: w662 -> [w671 w675]
            tunnel: w661 -> [_ w674]
            tunnel: w660 -> [w670 w673]
            tunnel: [w669 w672] -> w659
            frame False {
              n396 = Build Array (concatenate)(w671, w670) -> (w669:u32[][])
            }
            frame True {
              n397 = Replace Array Subset(array=w675, new element=w673, index (row)=w674) -> (w672:u32[][])  [unwired: 1 in]
            }
          }
        }
        frame True {
          n398 = local write "clear"(FALSE ("clear")) -> ()
          n399 = Build Array (concatenate)(u32[][] [] ("can_log"), w678) -> (w677:u32[][])
        }
      }
      n400 = case shown="True" "sortbyID" {
        tunnel: [w618 w621] -> w608
        tunnel: w609 -> [w618 w647]
        frame False {
        }
        frame True {
          n401 = Index Array(array=w647, index (col) #1=0 ("disabled index (col)"), index (col) #2=0 ("index (col)")) -> (element #1=w644:u32[], element #2=w643:u32[], element #3=w642:u32[], element #4=w641:u32[], element #5=w640:u32[], element #6=w639:u32[], element #7=w638:u32[], element #8=w637:u32[], element #9=w636:u32[], element #10=w635:u32[], element #11=w634:u32[])  [unwired: 20 in]
          n402 = local write "sortbyID"(FALSE ("sortbytime")) -> ()
          n403 = Build Cluster Array(w644, w643, w642, w641, w640, w639, w638, w637, w636, w635, w634) -> (w633:T2)
          n404 = Sort 1D Array(array=w633) -> (sorted array=w619:T2)
          n405 = for {
            tunnel: w619 -> [w658] mode=indexing
            tunnel: [w657] -> w632 mode=indexing
            tunnel: [w656] -> w631 mode=indexing
            tunnel: [w655] -> w630 mode=indexing
            tunnel: [w654] -> w629 mode=indexing
            tunnel: [w653] -> w628 mode=indexing
            tunnel: [w652] -> w627 mode=indexing
            tunnel: [w651] -> w626 mode=indexing
            tunnel: [w650] -> w625 mode=indexing
            tunnel: [w649] -> w624 mode=indexing
            tunnel: [w648] -> w623 mode=indexing
            n406 = Unbundle(w658) -> ("identifier"=w657:u32, "identifier"=w656:u32, "identifier"=w655:u32, "identifier"=w654:u32, "identifier"=w653:u32, "identifier"=w652:u32, "identifier"=w651:u32, "identifier"=w650:u32, "identifier"=w649:u32, "identifier"=w648:u32)  [unwired: 1 out]
          }
          n407 = Build Array(w632, w631, w630, w629, w628, w627, w626, w625, w624, w623) -> (w622:u32[][])
          n408 = Transpose 2D Array(2D array=w622) -> (transposed array=w621:u32[][])
        }
      }
      "can_log" <- w608
    }
  }
